vi "MsgParser.vi"(2 "Result Output Msg Table":string[][](table), 3 "Output VOC Msg LOG":string[][](table)=[["CODE", "PARAM"]], 4 "MSG Counter":i32, 5 "current msg num":i32) -> (0 "Result Counter":i32, 1 "Output Alg Msg":string[][](table))   [LabVIEW 2010]
panel:
  out "Result Output Msg Table 2":string[][](array[string])
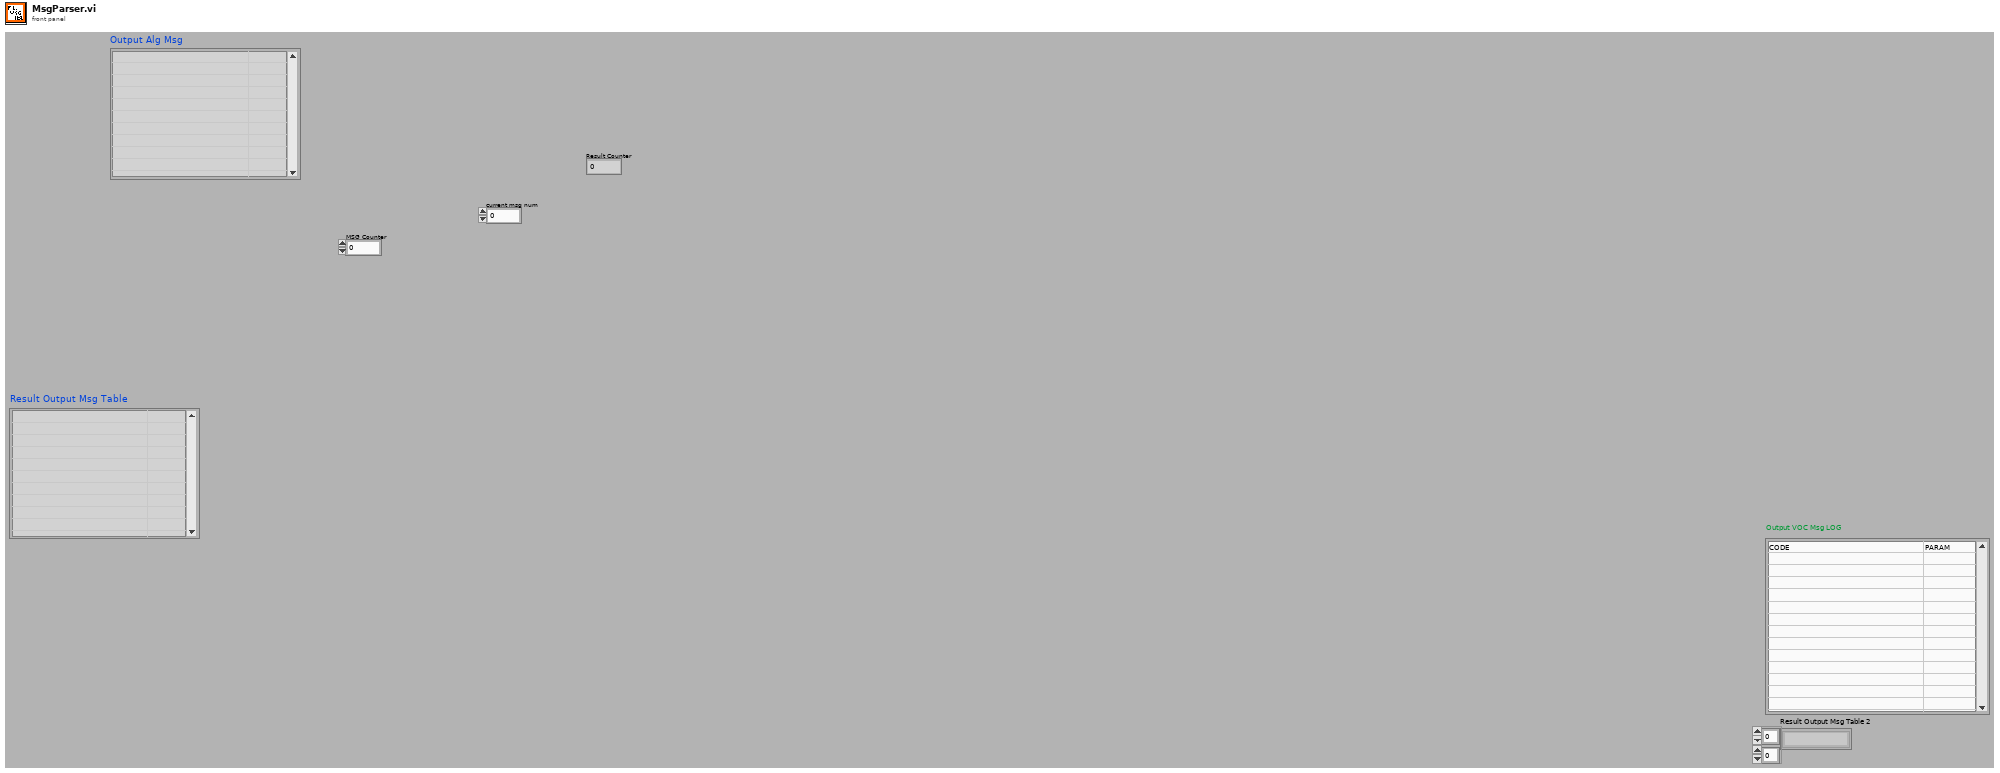
[diagram p1: front panel]
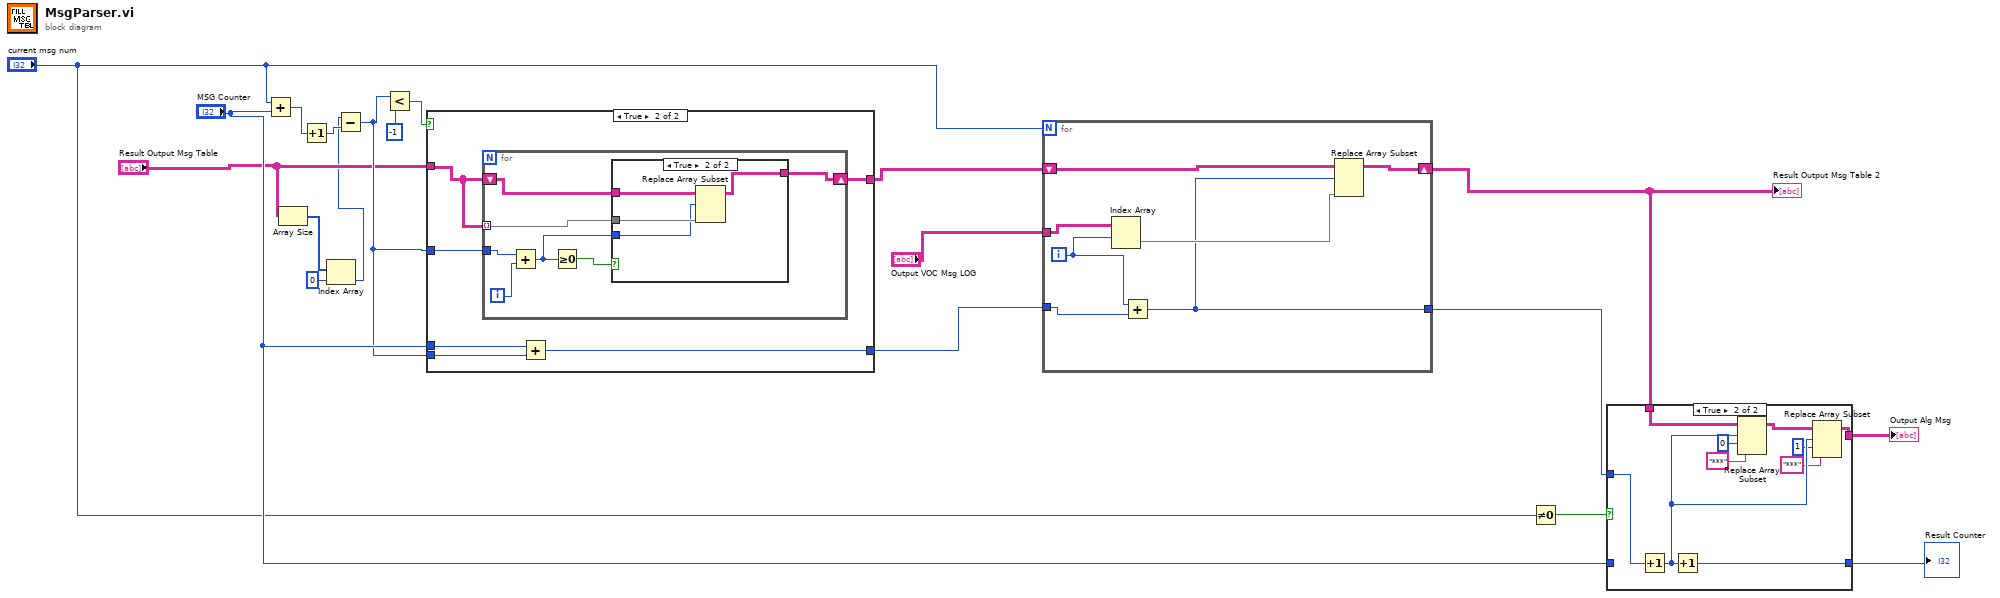
[diagram p0: block diagram]
diagram:
  n1 = Add(x="current msg num", y="MSG Counter") -> (x+y=w15:i32)
  n2 = Array Size(array="Result Output Msg Table") -> (size(s)=w3:i32[])
  n3 = Increment(x=w15) -> (x+1=w14:i32)
  n4 = Index Array(array=w3, index=0) -> (element=w1:i32)
  n5 = Subtract(x=w1, y=w14) -> (x-y=w13:i32)
  n6 = Less?(x=w13, y=-1) -> (x < y?=w11:bool)
  n7 = case shown="True" w11 {
    tunnel: "Result Output Msg Table" -> [w21 w27]
    tunnel: w13 -> [_ w26]
    tunnel: w13 -> [_ w23]
    tunnel: [w21 w25] -> w10
    tunnel: "MSG Counter" -> [w20 w24]
    tunnel: [w20 w22] -> w6
    frame False {
    }
    frame True {
      n8 = for {
        shift-right: [w32] -> w25
        shift-left: w27 -> [w34]
        tunnel: w27 -> [w33] mode=indexing
        tunnel: w26 -> [w31]
        i -> [w29]
        n9 = Add(x=w31, y=w29) -> (x+y=w28:i32)
        n10 = Greater Or Equal To 0?(x=w28) -> (x >= 0?=w30:bool)
        n11 = case shown="True" w30 {
          tunnel: w34 -> [w35 w39]
          tunnel: w33 -> [_ w38]
          tunnel: [w35 w37] -> w32
          tunnel: w28 -> [_ w36]
          frame False {
          }
          frame True {
            n12 = Replace Array Subset(array=w39, new element=w38, index (row)=w36) -> (w37:string[][])  [unwired: 1 in]
          }
        }
      }
      n13 = Add(x=w24, y=w23) -> (x+y=w22:i32)
    }
  }
  n14 = for {
    N: "current msg num" -> [_]
    shift-right: [w45] -> w9
    shift-left: w10 -> [w46]
    tunnel: "Output VOC Msg LOG" -> [w44]
    tunnel: w6 -> [w41]
    tunnel: [w40] -> w5
    i -> [w42]
    n15 = Index Array(array=w44, index (row)=w42) -> (element=w43:string[])  [unwired: 1 in]
    n16 = Add(x=w42, y=w41) -> (x+y=w40:i32)
    n17 = Replace Array Subset(array=w46, new element=w43, index (row)=w40) -> (w45:string[][])  [unwired: 1 in]
  }
  "Result Output Msg Table 2" <- w9
  n18 = Not Equal To 0?(x="current msg num") -> (x != 0?=w17:bool)
  n19 = case shown="True" w17 {
    tunnel: w5 -> [_ w58]
    tunnel: w9 -> [w48 w57]
    tunnel: [w48 w50] -> w19
    tunnel: [w47 w49] -> w18
    tunnel: "MSG Counter" -> [w47 _]
    frame False {
    }
    frame True {
      n20 = Increment(x=w58) -> (x+1=w55:i32)
      n21 = Increment(x=w55) -> (x+1=w49:i32)
      n22 = Replace Array Subset(array=w57, new element="***" ("new element/subarray"), index (row)=w55, index (col)=0 ("disabled index (col)")) -> (w56:string[][])
      n23 = Replace Array Subset(array=w56, new element="***" ("new element/subarray"), index (row)=w55, index (col)=1 ("disabled index (col)")) -> (w50:string[][])
    }
  }
  "Output Alg Msg" <- w19
  "Result Counter" <- w18
